vi "Get Waveform.vi"(8 "error in (no error)":errorcluster, 10 "Number of points":i32, 11 "RP Transceiver in":refnum<class "RP Transceiver.lvclass">) -> (0 "error out":errorcluster, 2 "Data out":i16[](array[numeric]), 3 "RP Transceiver out":refnum<class "RP Transceiver.lvclass">)   [LabVIEW 2015, in "RP Transceiver.lvclass"]
uses:
  RP Transceiver.lvclass
  RP Transceiver.lvclass/RP Transceiver.ctl
  RP Communicator/RP Communicator.lvclass
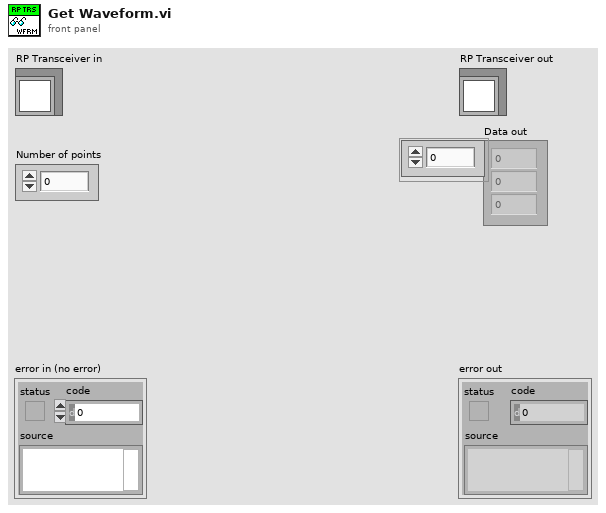
[diagram p1: front panel]
types:
  T1 = enum16{"big-endian, network order", "native, host order", "little-endian"}
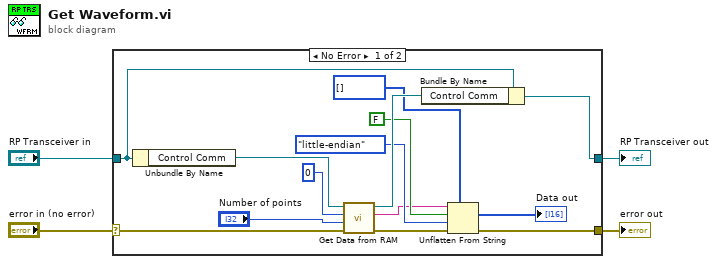
[diagram p0: block diagram]
diagram:
  n1 = case shown="No Error" "error in (no error)" {
    selector: "error in (no error)" -> [w16 w20]
    tunnel: [w7 w20] -> w3
    tunnel: [w13 w19] -> w1
    tunnel: "RP Transceiver in" -> [w18 w19]
    frame No Error {
      n2 = Unbundle By Name(w18) -> ("Control Comm"=w17:refnum<class "RP Communicator.lvclass">)
      n3 = call-dynamic "Get Data from RAM.vi"("error in (no error)"=w16, "End offset"="Number of points", "Start offset"=u64 0, "RP Communicator in"=w17) -> ("error out"=w8:errorcluster, "data out"=w6:string, "RP Communicator out"=w12:refnum<class "RP Communicator.lvclass">)  [unwired: 5 in]
      n4 = Bundle By Name(cluster=w18, "Control Comm"=w12) -> (w13:refnum<class "RP Transceiver.lvclass">)
      n5 = Unflatten From String(type=i16[] [], binary string=w6, data includes array or string size? (T)=FALSE, byte order (0:big-endian, network order)=T1."little-endian", error in (no error)=w8) -> (value=→"Data out":i16[], error out=w7:errorcluster)  [unwired: 1 out]
    }
    frame Error {
    }
  }
  "error out" <- w3
  "RP Transceiver out" <- w1
